vi "探头模板-16-20-网络版.vi"(11 "探头序号":T11(ring) caption="探头地址") -> ()   [LabVIEW 2017]
panel:
  out "初始尺寸":T1
  in  "报警方式[]":string[](array[string])
  out "报警方式a":T2
  out "探头状态a":T3
  out "累积":string="累积剂量/限值："
  in  "探头属性":T4={"探头地址与信息"={"网络地址"="", "名称"="", "备注"="", "累积剂量"=0.0, "累积限值"=0.0, "硬件剂量率限值"=enum."一级限值", "剂量率限值1"=0.0, "剂量率限值2"=0.0, "报警方式"=enum."常报警"}, "测量值"={"时间"=timestamp(3554955153.6246996 s since 1904-01-01), "数值"=0.0}, "限值"={"限值1"=0.0, "限值2"=0.0, "探头限值"=enum."一级限值"}, "探头状态"=enum."正常", "累积记录"={"起始时间"=timestamp(0 s since 1904-01-01), "结束时间"=timestamp(0 s since 1904-01-01), "累积剂量"=0.0}, "报警方式"={"报警方式"=enum."常报警", "延迟计时"=0, "报警中？"=FALSE}}
  in  "停止":bool=TRUE
  out "探头地址":T11(ring)
  out "探头信息":string
  in  "显示限值？":bool=TRUE
  out "测量值":dbl format="%.2g"
  out "探头状态":enum16{"正常", "离线", "禁用", "一级报警", "二级报警", "累积报警"}(ring)=enum."禁用"
  out "单位":enum16{"μSv/h", "mSv/h"}(ring)
  out "限值1":string="一级限值："
  out "限值2":string="二级限值："
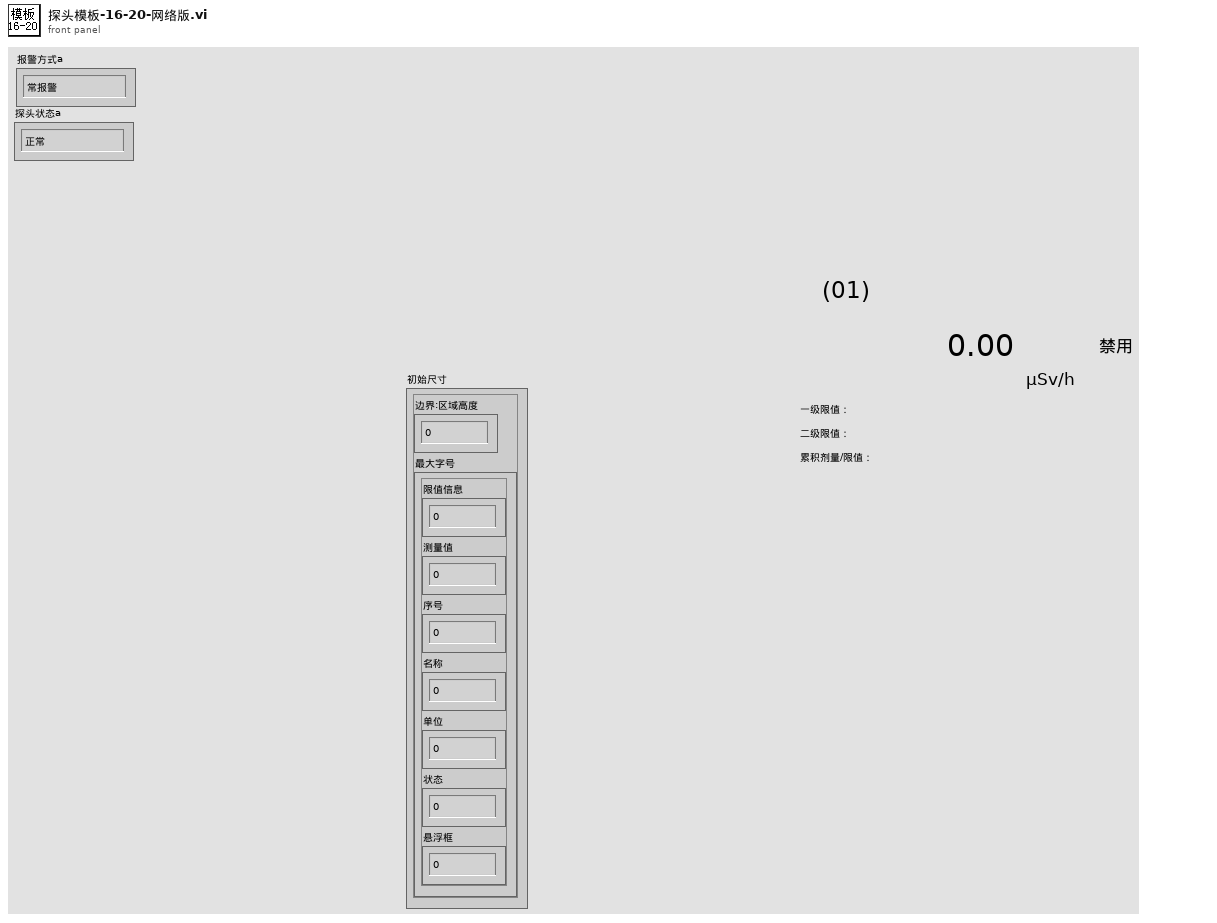
[diagram p1: front panel]
types:
  T1 = typedef "簇-界面模板初始字号.ctl" = cluster{"边界:区域高度":u32, "最大字号":cluster{"限值信息":u32, "测量值":u32, "序号":u32, "名称":u32, "单位":u32, "状态":u32, "悬浮框":u32}}
  T2 = typedef "报警方式选择.ctl" = enum16{"常报警", "自动静音", "手动静音"}
  T3 = typedef "探头状态.ctl" = enum16{"正常", "离线", "禁用", "一级报警", "二级报警", "累积报警"}
  T4 = typedef "探头属性.ctl" = cluster{"探头地址与信息":T5, "测量值":T7, "限值":T8, "探头状态":T3, "累积记录":T9, "报警方式":T10}
  T5 = typedef "探测器信息.ctl" = cluster{"网络地址":string, "名称":string, "备注":string, "累积剂量":dbl, "累积限值":dbl, "硬件剂量率限值":T6, "剂量率限值1":dbl, "剂量率限值2":dbl, "报警方式":T2}
  T6 = typedef "探头剂量率限值选择.ctl" = enum16{"一级限值", "二级限值"}
  T7 = typedef "测量值.ctl" = cluster{"时间":timestamp, "数值":dbl}
  T8 = typedef "剂量率限值.ctl" = cluster{"限值1":dbl, "限值2":dbl, "探头限值":T6}
  T9 = typedef "单条累积记录.ctl" = cluster{"起始时间":timestamp, "结束时间":timestamp, "累积剂量":dbl}
  T10 = typedef "报警方式.ctl" = cluster{"报警方式":T2, "延迟计时":u16, "报警中？":bool}
  T11 = enum16{"(01)", "(02)", "(03)", "(04)", "(05)", "(06)", "(07)", "(08)", "(09)", "(10)", "(11)", "(12)", "(13)", "(14)", "(15)", "(16)", "(17)", "(18)", "(19)", "(20)", "(21)", "(22)", "(23)", "(24)", "(25)", "(26)", "(27)", "(28)", "(29)", "(30)", "(31)", "(32)", "(33)", "(34)", "(35)"}
  T12 = cluster{"限值信息":u32, "测量值":u32, "序号":u32, "名称":u32, "单位":u32, "状态":u32, "悬浮框":u32}
  T13 = enum8{"Enabled", "Disabled", "Disabled and Grayed Out"}
  T14 = cluster{"原始尺寸":cluster{"所在窗格高度":u32, "字号":u32}, "new所在窗格高度":u32}
  T15 = enum16{"No Scaling", "Scale All Objects", "Scale Single Object"}
  T16 = typedef "LVRectTypeDef.ctl" = cluster{"Left":i16, "Top":i16, "Right":i16, "Bottom":i16}
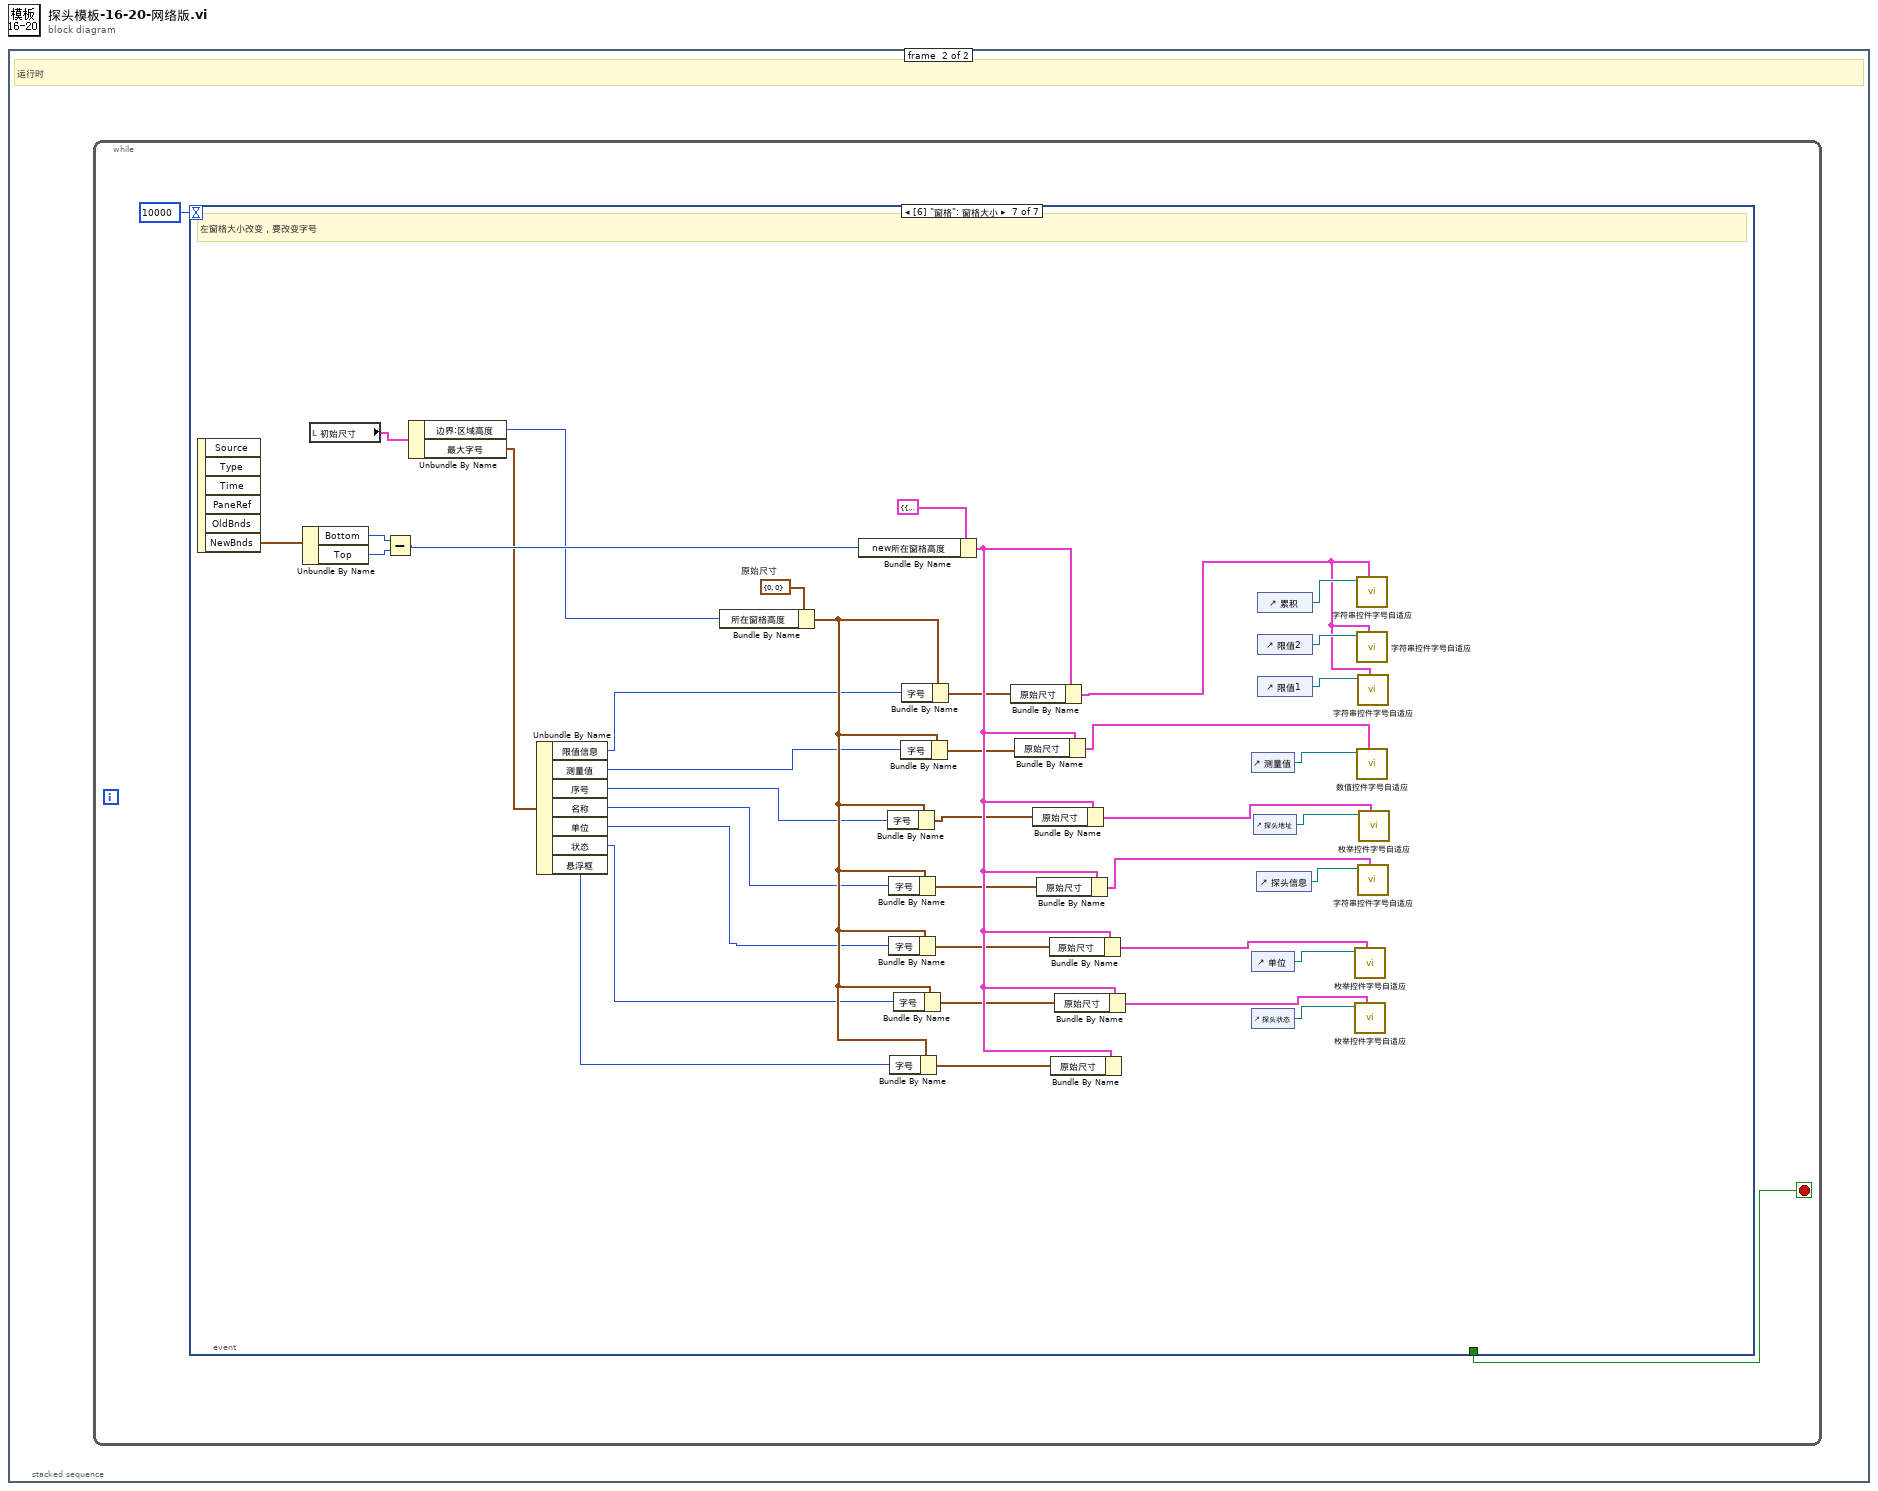
[diagram p0: block diagram]
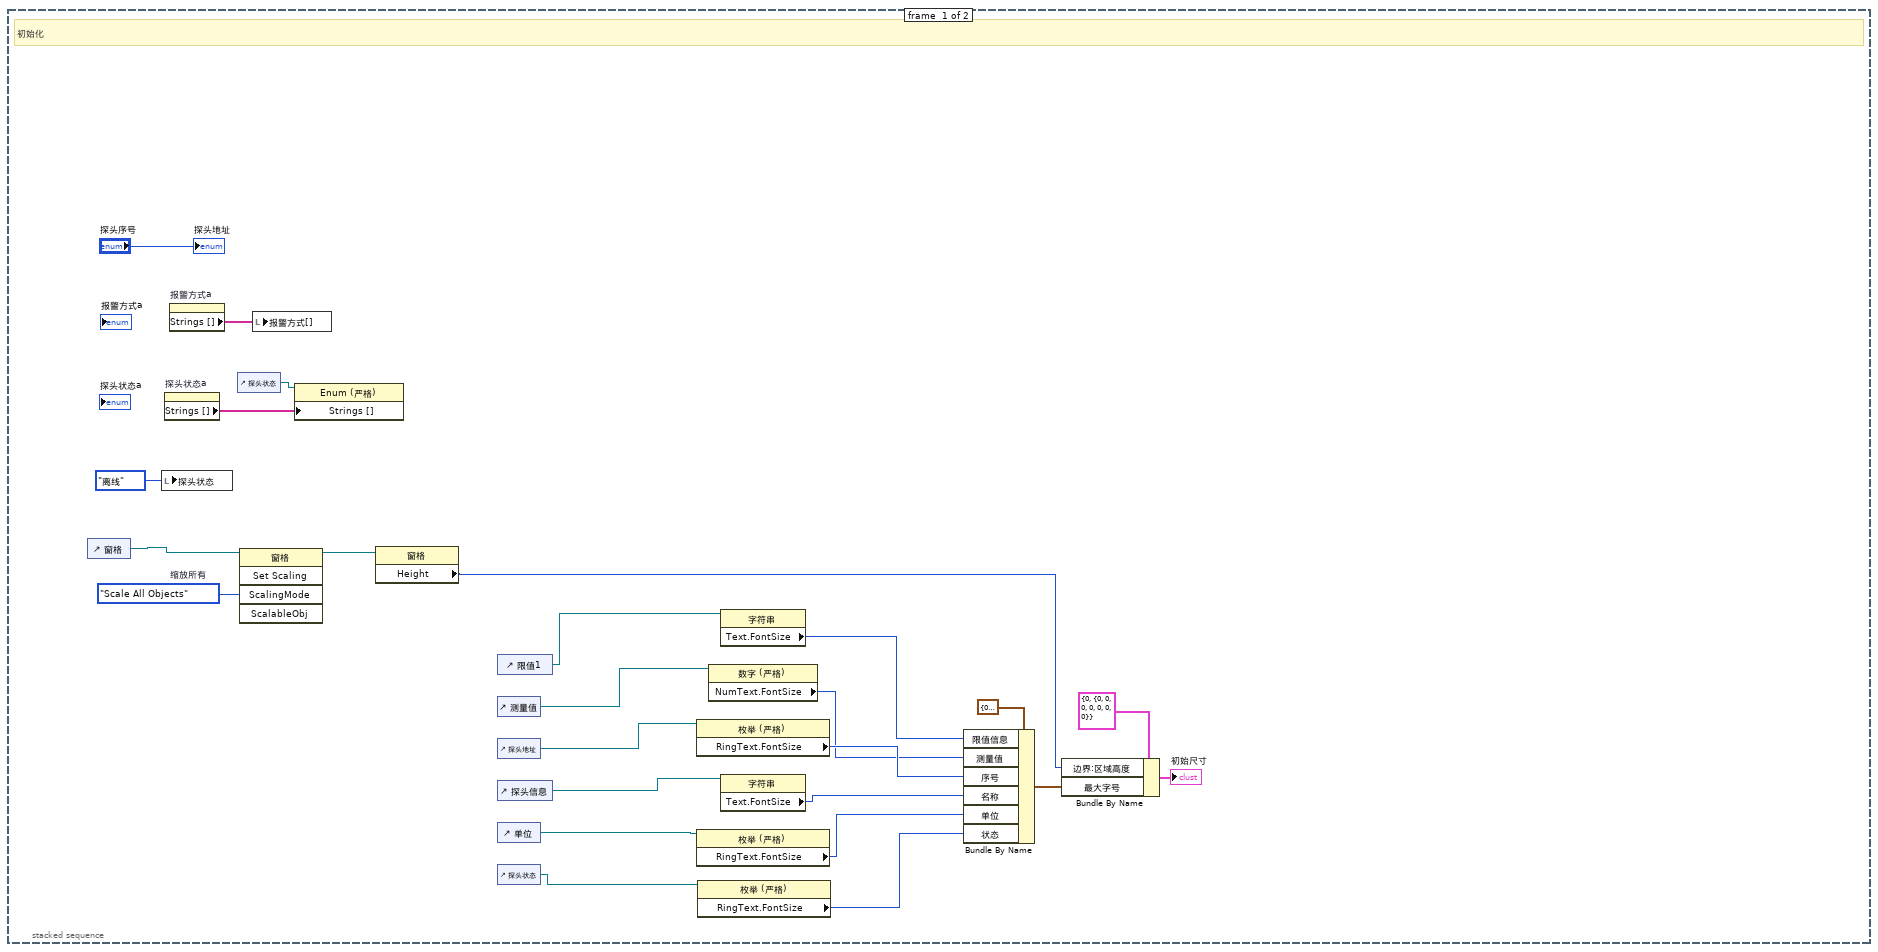
[diagram p2: hidden frame]
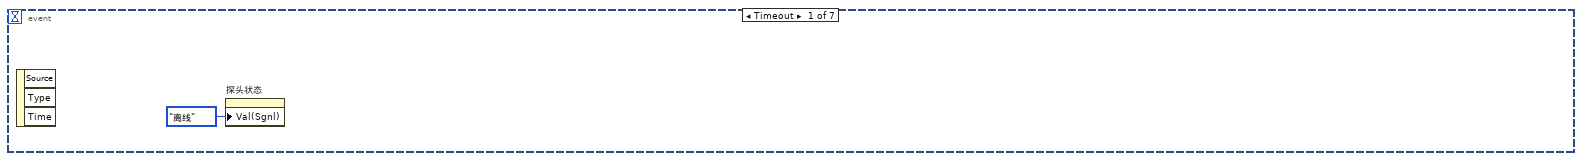
[diagram p3: hidden frame]
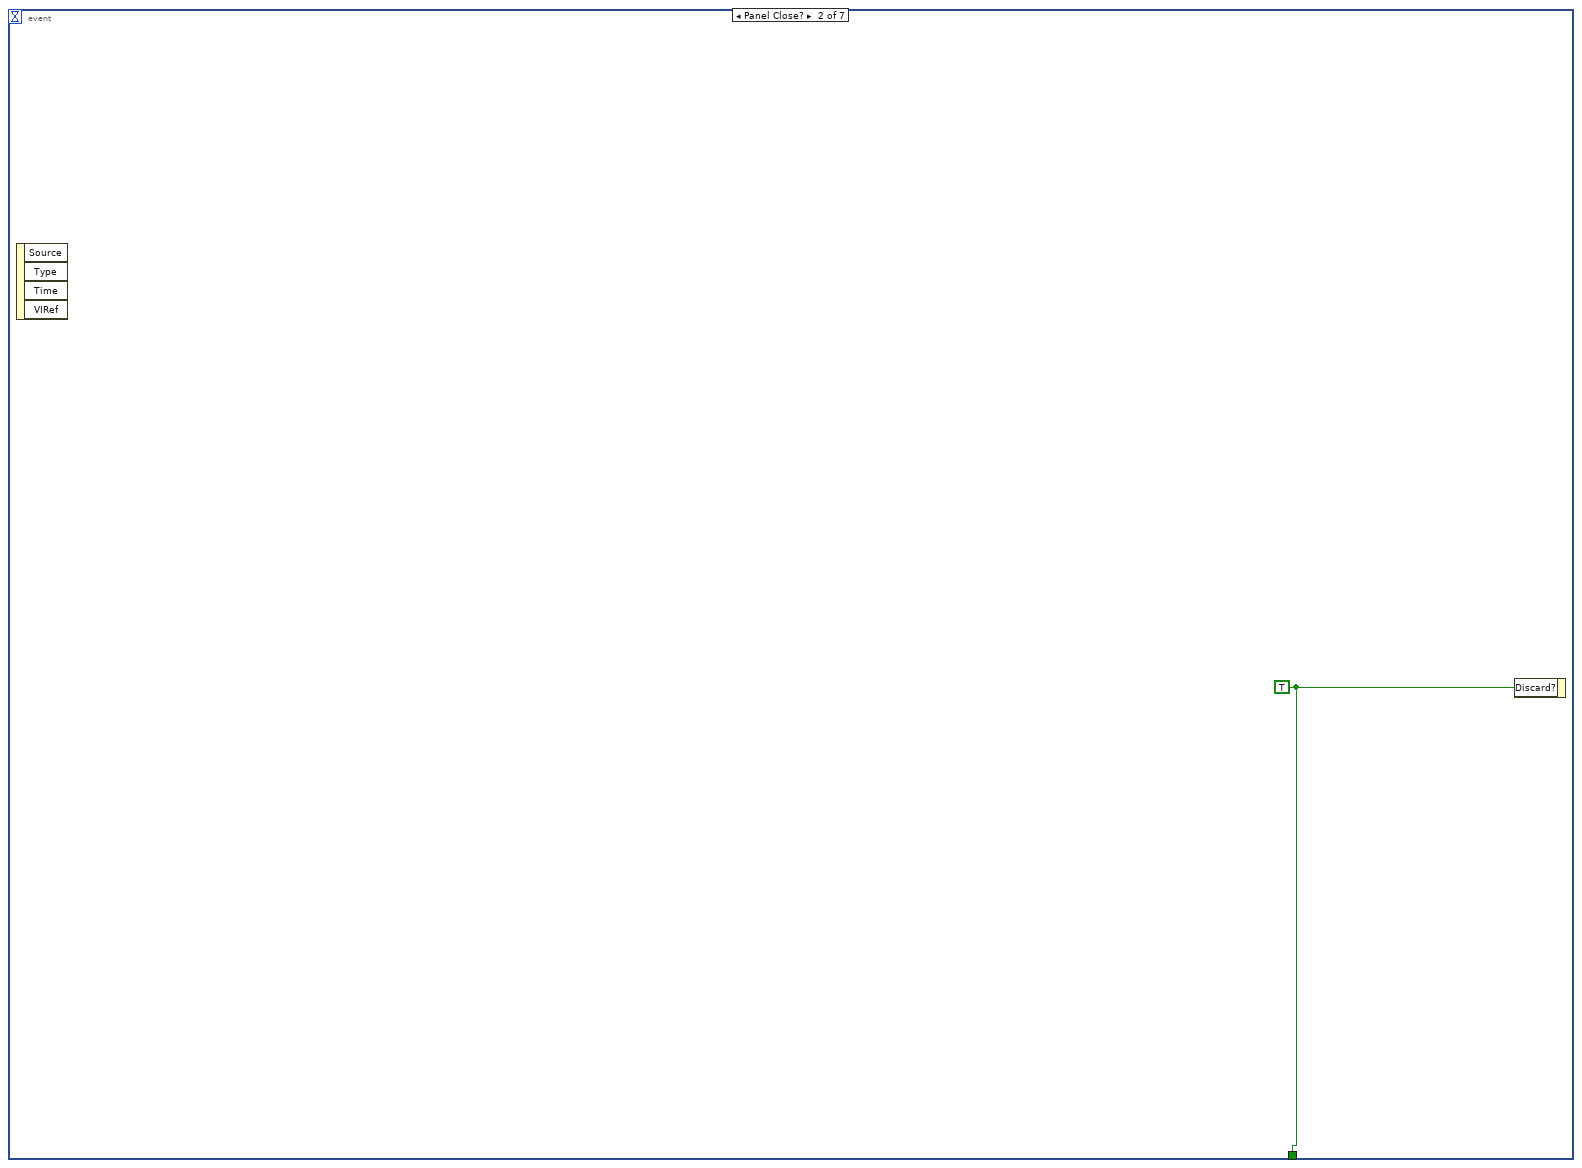
[diagram p4: hidden frame]
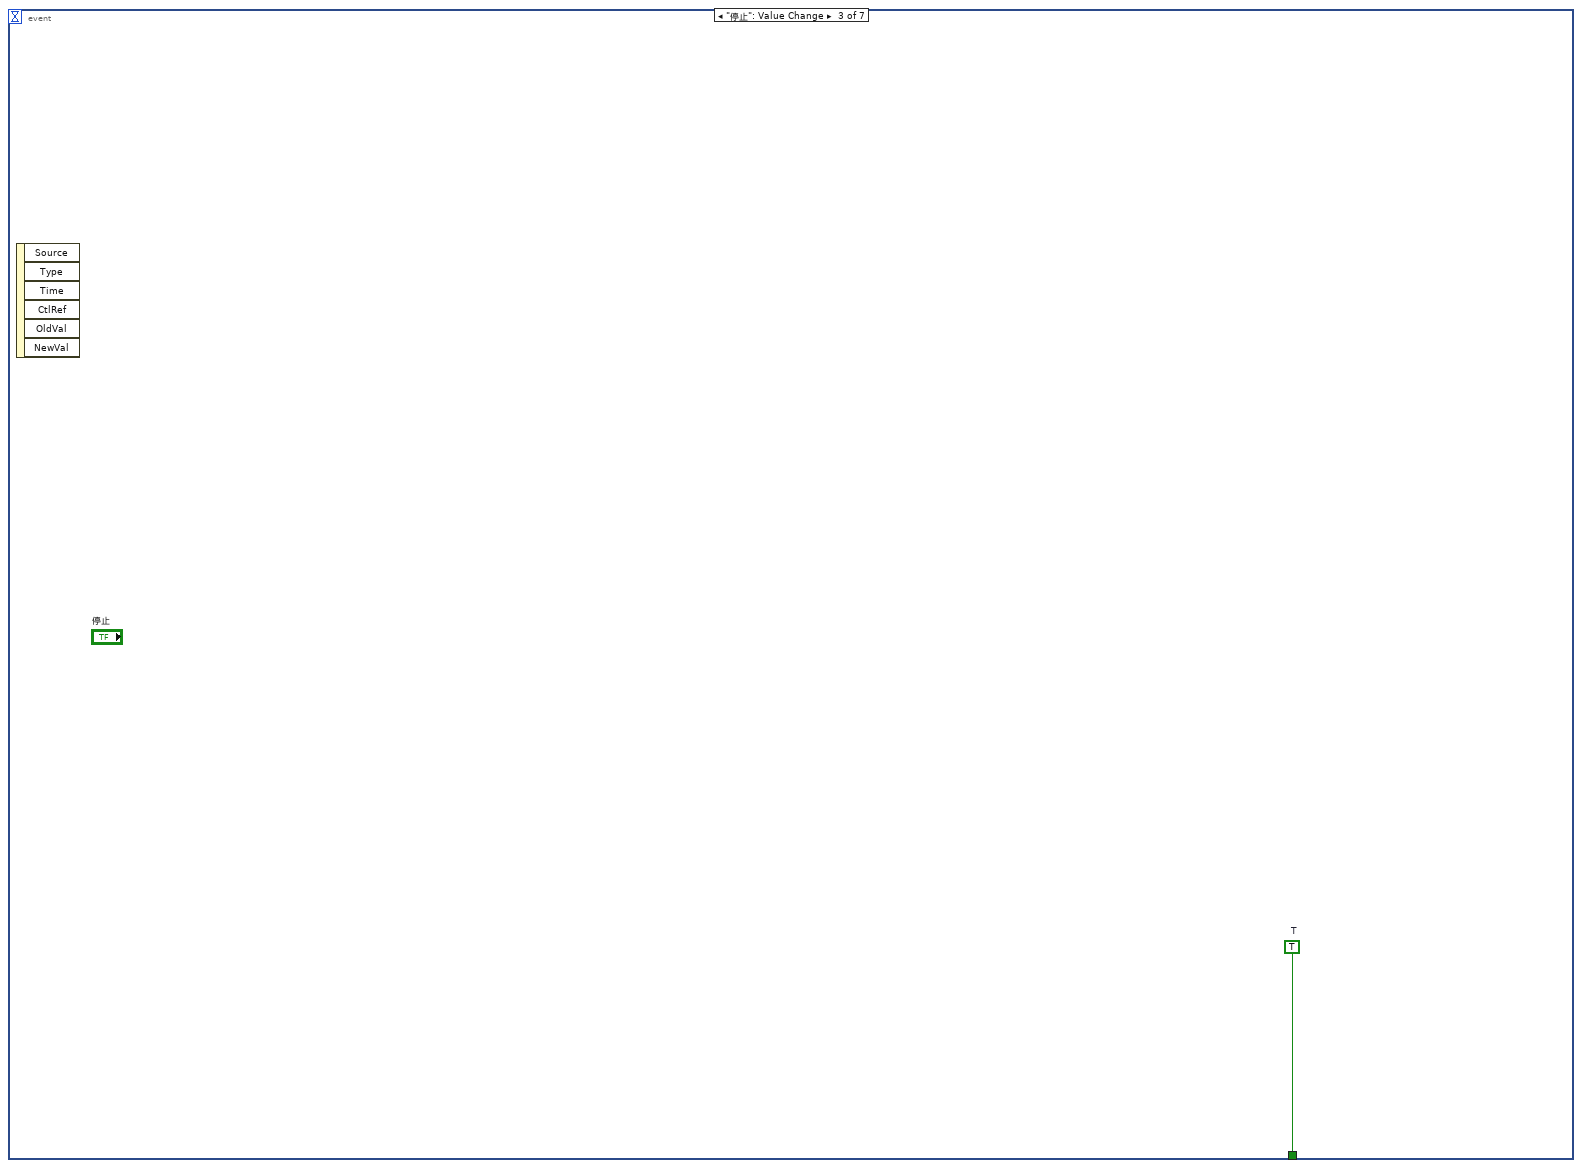
[diagram p5: hidden frame]
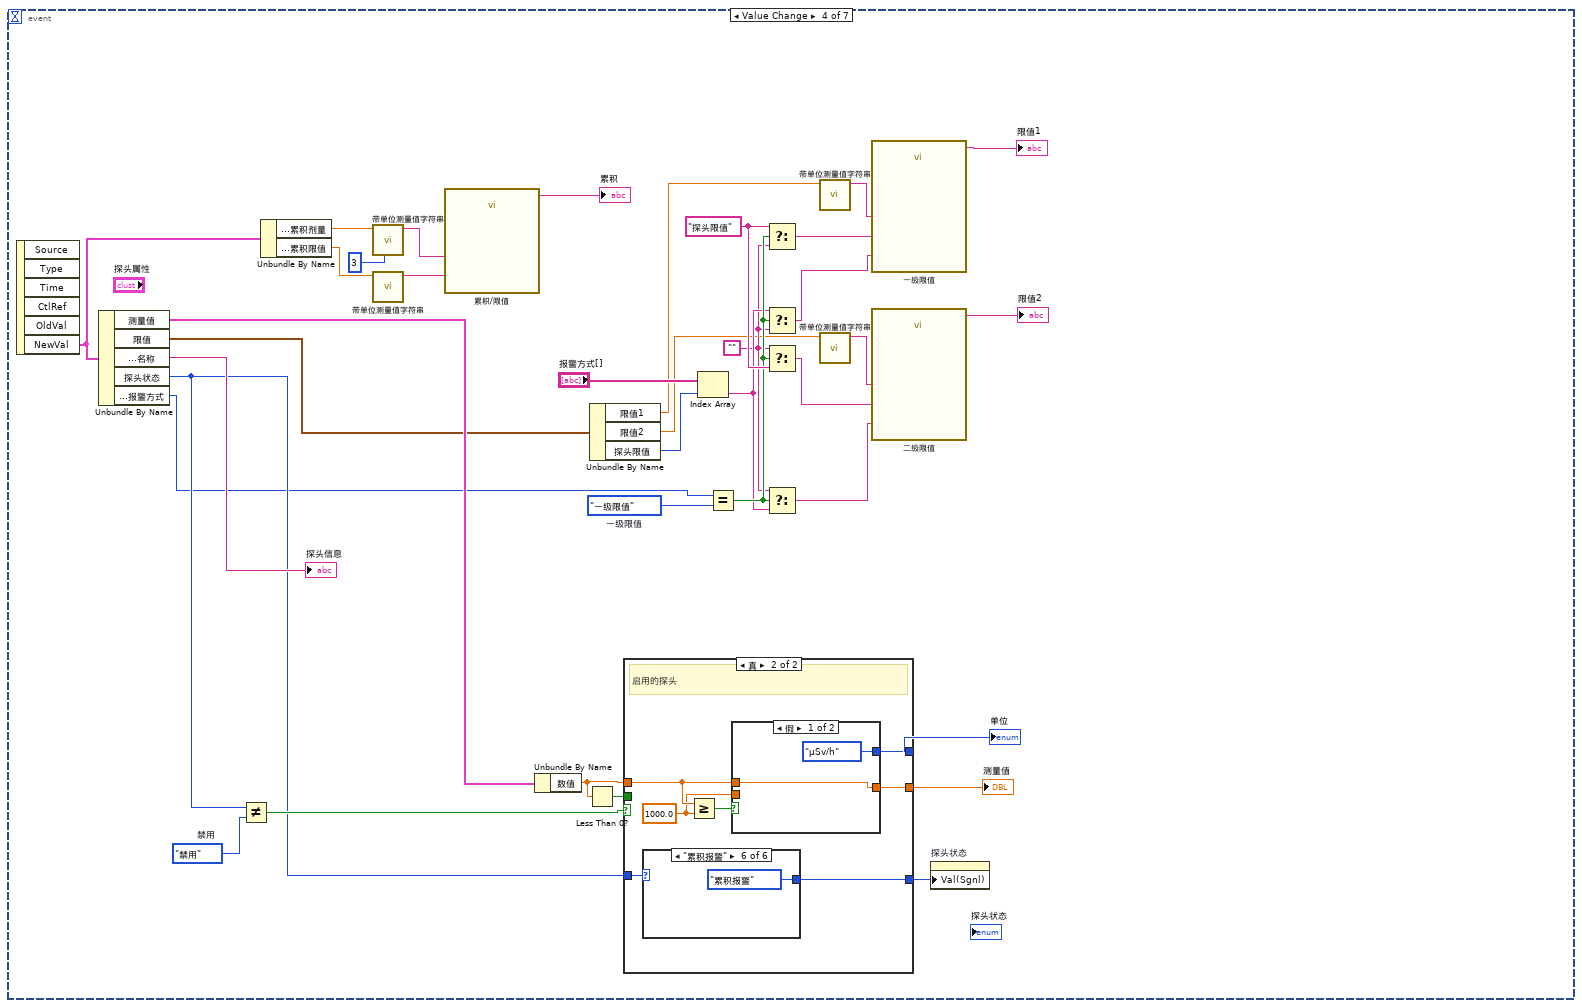
[diagram p6: hidden frame]
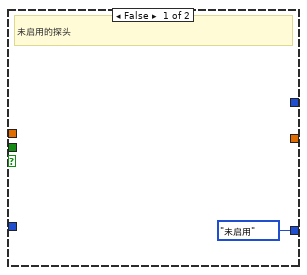
[diagram p7: hidden frame]
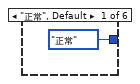
[diagram p8: hidden frame]
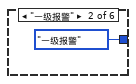
[diagram p9: hidden frame]
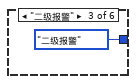
[diagram p10: hidden frame]
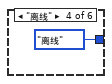
[diagram p11: hidden frame]
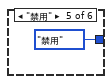
[diagram p12: hidden frame]
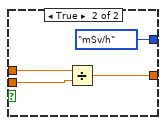
[diagram p13: hidden frame]
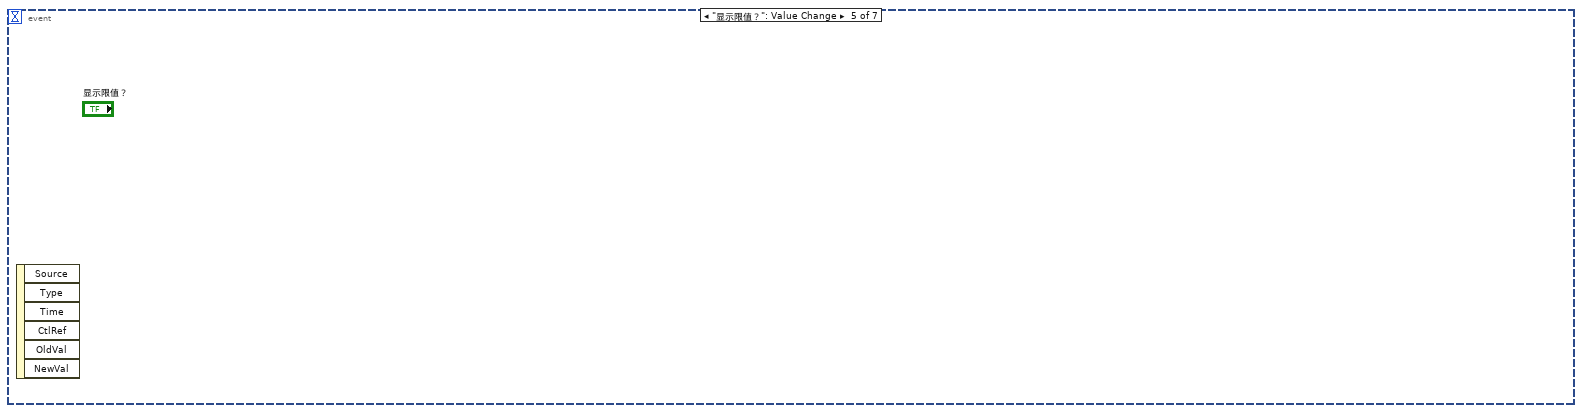
[diagram p14: hidden frame]
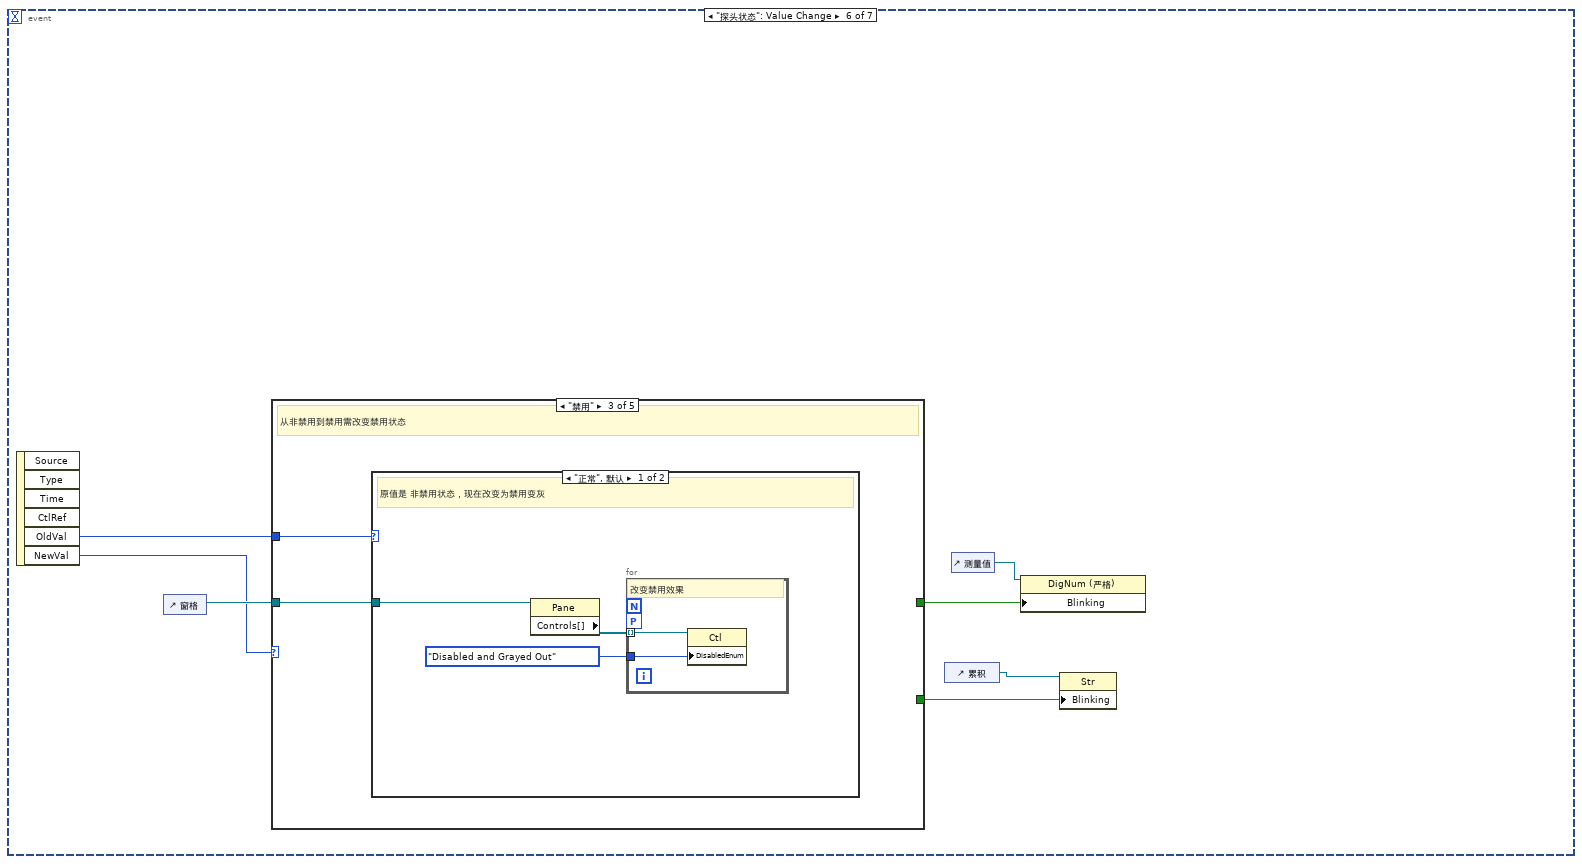
[diagram p15: hidden frame]
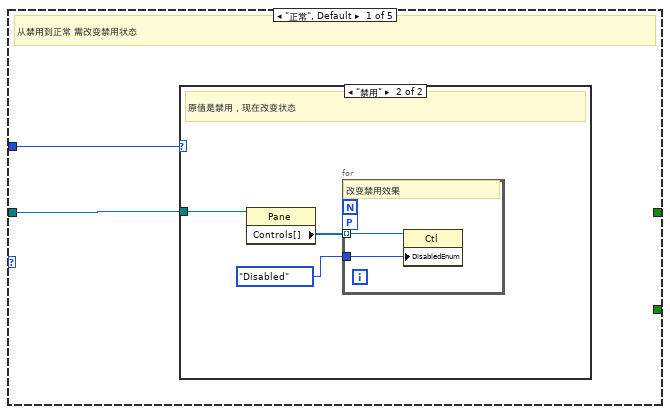
[diagram p16: hidden frame]
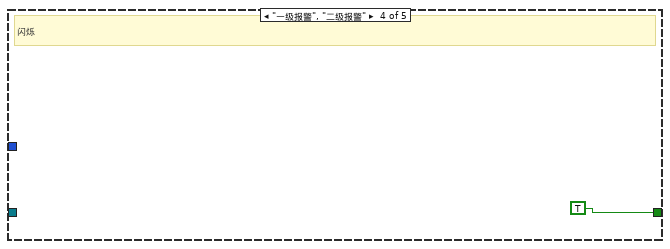
[diagram p20: hidden frame]
diagram:
  n1 = stacked-sequence {
    frame #0 {
      w19 = T15."Scale All Objects"  # 缩放所有
      # "初始化"
      n2 = control-ref of="窗格"() -> (w18:refnum<vi>)
      n3 = local write "探头状态"(探头状态."离线" ("探头状态")) -> ()
      n4 = property on="探头状态a" class="Enum (严格)"() -> ("Strings []"=w22:string[])  [unwired: 2 in, 2 out]
      n5 = property on="报警方式a" class="Enum (严格)"() -> ("Strings []"=w21:string[])  [unwired: 2 in, 2 out]
      n6 = control-ref of="探头状态"() -> (w23:refnum<vi>)
      n7 = invoke class="窗格" method="Set Scaling"(reference=w18, "ScalingMode"=w19) -> (reference out=w20:refnum<vi>)  [unwired: 3 in, 4 out]
      n8 = local write "报警方式[]"(w21) -> ()
      n9 = property on="属性节点" class="Enum (严格)"(reference=w23, "Strings []"=w22) -> ()  [unwired: 1 in, 2 out]
      n10 = property class="窗格"(reference=w20) -> ("Height"=w7:u32)  [unwired: 1 in, 2 out]
      n11 = control-ref of="限值1"() -> (w6:refnum<vi>)
      n12 = control-ref of="测量值"() -> (w5:refnum<vi>)
      n13 = control-ref of="探头地址"() -> (w4:refnum<vi>)
      n14 = control-ref of="探头信息"() -> (w3:refnum<vi>)
      n15 = control-ref of="单位"() -> (w2:refnum<vi>)
      n16 = control-ref of="探头状态"() -> (w1:refnum<vi>)
      n17 = property class="枚举 (严格)"(reference=w4) -> ("RingText.FontSize"=w14:u32)  [unwired: 1 in, 2 out]
      n18 = property class="枚举 (严格)"(reference=w2) -> ("RingText.FontSize"=w16:u32)  [unwired: 1 in, 2 out]
      n19 = property class="枚举 (严格)"(reference=w1) -> ("RingText.FontSize"=w17:u32)  [unwired: 1 in, 2 out]
      n20 = property class="数字 (严格)"(reference=w5) -> ("NumText.FontSize"=w13:u32)  [unwired: 1 in, 2 out]
      n21 = property class="字符串"(reference=w6) -> ("Text.FontSize"=w12:u32)  [unwired: 1 in, 2 out]
      n22 = property class="字符串"(reference=w3) -> ("Text.FontSize"=w15:u32)  [unwired: 1 in, 2 out]
      n23 = Bundle By Name(cluster=T12 {"限值信息"=0, "测量值"=0, "序号"=0, "名称"=0, "单位"=0, "状态"=0, "悬浮框"=0} ("最大字号"), "限值信息"=w12, "测量值"=w13, "序号"=w14, "名称"=w15, "单位"=w16, "状态"=w17) -> (w8:T12)
      n24 = Bundle By Name(cluster=T1 {"边界:区域高度"=0, "最大字号"={"限值信息"=0, "测量值"=0, "序号"=0, "名称"=0, "单位"=0, "状态"=0, "悬浮框"=0}} ("输出簇"), "边界:区域高度"=w7, "最大字号"=w8) -> (→"初始尺寸":T1)
      "探头地址" <- "探头序号"
    }
    frame #1 {
      # "运行时"
      n25 = while {
        stop <- w27 stop-if-true
        n26 = event shown="[6] \"窗格\": 窗格大小" {
          selector: _ -> [_ _ _ _ _ _ _]
          dyn-events: _ -> [_ _ _ _ _ _ _]
          timeout: 10000 -> [_ _ _ _ _ _ _]
          tunnel: [_ w29 w30 _ _ _ _] -> w27
          event Timeout {
            n27 = event-data() -> ()  [unwired: 1 in, 3 out]
            n28 = property on="探头状态" class="Enum (严格)"("Val(Sgnl)"=探头状态."离线" ("值(信号)")) -> ()  [unwired: 2 in, 2 out]
          }
          event Panel Close? {
            w29 = TRUE ("放弃？")
            n29 = event-data() -> ()  [unwired: 1 in, 4 out]
            n30 = event-data("Discard?"=w29) -> ()  [unwired: 1 in, 1 out]
          }
          event "停止": Value Change {
            w30 = TRUE  # T
            n31 = event-data() -> ()  [unwired: 1 in, 6 out]
          }
          event Value Change {
            w47 = ""
            w50 = "探头限值" ("F-格式字符串")
            w51 = 探头剂量率限值选择."一级限值"  # 一级限值
            w61 = 探头状态."禁用"  # 禁用
            n32 = event-data() -> ("NewVal"=w52:T4)  [unwired: 1 in, 5 out]
            n33 = Unbundle By Name(w52) -> ("测量值"=w60:T7, "限值"=w59:T8, "探头地址与信息.名称"=→"探头信息":string, "探头状态"=w56:T3, "探头地址与信息.报警方式"=w40:T2)
            n34 = Not Equal?(x=w56, y=w61) -> (x != y?=w57:bool)
            n35 = Unbundle By Name(w52) -> ("探头地址与信息.累积剂量"=w36:dbl, "探头地址与信息.累积限值"=w35:dbl)
            n36 = call "带单位测量值字符串.vi"("精度(2)"=i16 3, "测量值"=w36) -> ("结果"=w33:string)  [unwired: 9 in]
            n37 = call "带单位测量值字符串.vi"("测量值"=w35) -> ("结果"=w34:string)  [unwired: 10 in]
            n38 = call "累积/限值"("累积剂量"=w33, "累积限值"=w34) -> ("Result"=→"累积":string)  [unwired: 12 in, 1 out]
            n39 = Unbundle By Name(w60) -> ("数值"=w66:dbl)
            n40 = Less Than 0?(x=w66) -> (x < 0?=w65:bool)
            n41 = Unbundle By Name(w59) -> ("限值1"=w32:dbl, "限值2"=w38:dbl, "探头限值"=w45:T6)
            n42 = case shown="真" w57 {
              tunnel: w65 -> [_ _]
              tunnel: w66 -> [_ w74]
              tunnel: [_ w73] -> w64
              tunnel: [_ w72] -> w63
              tunnel: [enum16{"正常", "未启用", "离线", "一级报警", "二级报警"}."未启用" ("探头状态") w71] -> w62
              tunnel: w56 -> [_ w70]
              frame False {
                # "未启用的探头"
              }
              frame True {
                w68 = 1000.0 ("y")
                # "启用的探头"
                n43 = case shown="\"累积报警\"" w70 {
                  tunnel: [探头状态."正常" ("探头状态") 探头状态."一级报警" ("探头状态") 探头状态."二级报警" ("探头状态") 探头状态."离线" ("探头状态") 探头状态."禁用" ("探头状态") 探头状态."累积报警" ("探头状态")] -> w71
                  frame "正常", Default {
                  }
                  frame "一级报警" {
                  }
                  frame "二级报警" {
                  }
                  frame "离线" {
                  }
                  frame "禁用" {
                  }
                  frame "累积报警" {
                  }
                }
                n44 = Greater Or Equal?(x=w74, y=w68) -> (x >= y?=w69:bool)
                n45 = case shown="假" w69 {
                  tunnel: w74 -> [w82 w86]
                  tunnel: w68 -> [_ w85]
                  tunnel: [w82 w84] -> w73
                  tunnel: [enum16{"μSv/h", "mSv/h"}."μSv/h" ("单位") enum16{"μSv/h", "mSv/h"}."mSv/h" ("单位")] -> w72
                  frame False {
                  }
                  frame True {
                    n46 = Divide(x=w86, y=w85) -> (x/y=w84:dbl)
                  }
                }
              }
            }
            "测量值" <- w64
            "单位" <- w63
            n47 = Index Array(array="报警方式[]", index=w45) -> (element=w48:string)
            n48 = Equal?(x=w40, y=w51) -> (x = y?=w49:bool)
            n49 = Select(t=w50, s=w49, f=w47) -> (s? t:f=w44:string)
            n50 = Select(t=w48, s=w49, f=w47) -> (s? t:f=w42:string)
            n51 = Select(t=w47, s=w49, f=w50) -> (s? t:f=w43:string)
            n52 = Select(t=w47, s=w49, f=w48) -> (s? t:f=w41:string)
            n53 = call "带单位测量值字符串.vi"("测量值"=w32) -> ("结果"=w39:string)  [unwired: 10 in]
            n54 = call "带单位测量值字符串.vi"("测量值"=w38) -> ("结果"=w37:string)  [unwired: 10 in]
            n55 = call "一级限值"("一级限值"=w39, "说明"=w44, "报警方式"=w42) -> ("Result"=→"限值1":string)  [unwired: 11 in, 1 out]
            n56 = call "二级限值"("二级限值"=w37, "说明"=w43, "报警方式"=w41) -> ("Result"=→"限值2":string)  [unwired: 11 in, 1 out]
            n57 = property on="探头状态" class="Enum (严格)"("Val(Sgnl)"=w62) -> ()  [unwired: 2 in, 2 out]
          }
          event "显示限值？": Value Change {
            n58 = event-data() -> ()  [unwired: 1 in, 6 out]
          }
          event "探头状态": Value Change {
            n59 = event-data() -> ("OldVal"=w92:enum16{"正常", "离线", "禁用", "一级报警", "二级报警", "累积报警"}, "NewVal"=w91:enum16{"正常", "离线", "禁用", "一级报警", "二级报警", "累积报警"})  [unwired: 1 in, 4 out]
            n60 = control-ref of="窗格"() -> (w93:refnum<vi>)
            n61 = case shown="\"禁用\"" w91 {
              tunnel: w92 -> [w95 _ w102 _ _]
              tunnel: w93 -> [w94 _ w101 _ _]
              tunnel: [_ _ _ TRUE _] -> w88
              tunnel: [_ _ _ _ TRUE] -> w87
              frame "正常", Default {
                # "从禁用到正常 需改变禁用状态"
                n62 = case shown="\"禁用\"" w95 {
                  tunnel: w94 -> [_ w97]
                  frame "正常", Default {
                  }
                  frame "禁用" {
                    # "原值是禁用，现在改变状态"
                    n63 = property class="Pane"(reference=w97) -> ("Controls[]"=w98:refnum<vi>[])  [unwired: 1 in, 2 out]
                    n64 = for {
                      tunnel: w98 -> [w100] mode=indexing
                      workers-P: _ -> [_]
                      tunnel: T13."Disabled" ("禁用") -> [w99]
                      # "改变禁用效果"
                      n65 = property class="Ctl"(reference=w100, "DisabledEnum"=w99) -> ()  [unwired: 1 in, 2 out]
                    }
                  }
                }
              }
              frame "离线" {
                # "无需动作"
              }
              frame "禁用" {
                # "从非禁用到禁用需改变禁用状态"
                n66 = case shown="\"正常\", 默认" w102 {
                  tunnel: w101 -> [w104 _]
                  frame "正常", Default {
                    # "原值是 非禁用状态，现在改变为禁用变灰"
                    n67 = property class="Pane"(reference=w104) -> ("Controls[]"=w105:refnum<vi>[])  [unwired: 1 in, 2 out]
                    n68 = for {
                      tunnel: w105 -> [w107] mode=indexing
                      workers-P: _ -> [_]
                      tunnel: T13."Disabled and Grayed Out" ("禁用") -> [w106]
                      # "改变禁用效果"
                      n69 = property class="Ctl"(reference=w107, "DisabledEnum"=w106) -> ()  [unwired: 1 in, 2 out]
                    }
                  }
                  frame "禁用" {
                    # "原来就是禁用状态，不改变"
                  }
                }
              }
              frame "一级报警", "二级报警" {
                # "闪烁"
              }
              frame "累积报警" {
              }
            }
            n70 = control-ref of="累积"() -> (w90:refnum<vi>)
            n71 = control-ref of="测量值"() -> (w89:refnum<vi>)
            n72 = property class="DigNum (严格)"(reference=w89, "Blinking"=w88) -> ()  [unwired: 1 in, 2 out]
            n73 = property class="Str"(reference=w90, "Blinking"=w87) -> ()  [unwired: 1 in, 2 out]
          }
          event Pane Size {
            w125 = cluster{"所在窗格高度":u32, "字号":u32} {"所在窗格高度"=0, "字号"=0}  # 原始尺寸
            # "左窗格大小改变，要改变字号"
            n74 = event-data() -> ("NewBnds"=w138:T16)  [unwired: 1 in, 5 out]
            n75 = Unbundle By Name(w138) -> ("Bottom"=w140:i16, "Top"=w139:i16)
            n76 = local read "初始尺寸"() -> (w137:T1)
            n77 = Subtract(x=w140, y=w139) -> (x-y=w118:i16)
            n78 = Unbundle By Name(w137) -> ("边界:区域高度"=w117:u32, "最大字号"=w116:T12)
            n79 = Unbundle By Name(w116) -> ("限值信息"=w127:u32, "测量值"=w128:u32, "序号"=w129:u32, "名称"=w130:u32, "单位"=w131:u32, "状态"=w132:u32, "悬浮框"=w136:u32)
            n80 = Bundle By Name(cluster=w125, "所在窗格高度"=w117) -> (w135:cluster{"所在窗格高度":u32, "字号":u32})
            n81 = Bundle By Name(cluster=T14 {"原始尺寸"={"所在窗格高度"=0, "字号"=0}, "new所在窗格高度"=0} ("输出簇"), "new所在窗格高度"=w118) -> (w134:T14)
            n82 = Bundle By Name(cluster=w135, "字号"=w129) -> (w122:cluster{"所在窗格高度":u32, "字号":u32})
            n83 = Bundle By Name(cluster=w135, "字号"=w130) -> (w121:cluster{"所在窗格高度":u32, "字号":u32})
            n84 = Bundle By Name(cluster=w135, "字号"=w131) -> (w120:cluster{"所在窗格高度":u32, "字号":u32})
            n85 = Bundle By Name(cluster=w135, "字号"=w136) -> (w133:cluster{"所在窗格高度":u32, "字号":u32})
            n86 = Bundle By Name(cluster=w135, "字号"=w132) -> (w119:cluster{"所在窗格高度":u32, "字号":u32})
            n87 = Bundle By Name(cluster=w135, "字号"=w128) -> (w123:cluster{"所在窗格高度":u32, "字号":u32})
            n88 = Bundle By Name(cluster=w135, "字号"=w127) -> (w124:cluster{"所在窗格高度":u32, "字号":u32})
            n89 = Bundle By Name(cluster=w134, "原始尺寸"=w124) -> (w115:T14)
            n90 = Bundle By Name(cluster=w134, "原始尺寸"=w123) -> (w114:T14)
            n91 = Bundle By Name(cluster=w134, "原始尺寸"=w122) -> (w113:T14)
            n92 = Bundle By Name(cluster=w134, "原始尺寸"=w121) -> (w112:T14)
            n93 = Bundle By Name(cluster=w134, "原始尺寸"=w120) -> (w111:T14)
            n94 = Bundle By Name(cluster=w134, "原始尺寸"=w133) -> ()  [unwired: 1 out]
            n95 = Bundle By Name(cluster=w134, "原始尺寸"=w119) -> (w110:T14)
            n96 = control-ref of="测量值"() -> (w141:refnum<vi>)
            n97 = control-ref of="单位"() -> (w144:refnum<vi>)
            n98 = control-ref of="探头状态"() -> (w143:refnum<vi>)
            n99 = control-ref of="探头地址"() -> (w142:refnum<vi>)
            n100 = control-ref of="探头信息"() -> (w145:refnum<vi>)
            n101 = control-ref of="累积"() -> (w148:refnum<vi>)
            n102 = control-ref of="限值2"() -> (w147:refnum<vi>)
            n103 = control-ref of="限值1"() -> (w146:refnum<vi>)
            n104 = call "枚举控件字号自适应.vi"("新旧尺寸信息"=w111, "枚举控件-引用"=w144) -> ()  [unwired: 8 in, 2 out]
            n105 = call "枚举控件字号自适应.vi"("新旧尺寸信息"=w110, "枚举控件-引用"=w143) -> ()  [unwired: 8 in, 2 out]
            n106 = call "字符串控件字号自适应.vi"("新旧尺寸信息"=w115, "字符串控件-引用"=w148) -> ()  [unwired: 8 in, 2 out]
            n107 = call "字符串控件字号自适应.vi"("新旧尺寸信息"=w115, "字符串控件-引用"=w147) -> ()  [unwired: 8 in, 2 out]
            n108 = call "数值控件字号自适应.vi"("新旧尺寸信息"=w114, "数值控件-引用"=w141) -> ()  [unwired: 8 in, 2 out]
            n109 = call "字符串控件字号自适应.vi"("新旧尺寸信息"=w115, "字符串控件-引用"=w146) -> ()  [unwired: 8 in, 2 out]
            n110 = call "字符串控件字号自适应.vi"("新旧尺寸信息"=w112, "字符串控件-引用"=w145) -> ()  [unwired: 8 in, 2 out]
            n111 = call "枚举控件字号自适应.vi"("新旧尺寸信息"=w113, "枚举控件-引用"=w142) -> ()  [unwired: 8 in, 2 out]
          }
        }
      }
    }
  }
